vi "BuildRelease_FixAF2014.vi"(8 "error in (no error)":errorcluster, 11 "Array in":refnum<vi>[](array[refnum])) -> (0 "error out":errorcluster, 3 "Array out":refnum<vi>[](array[refnum]))   [LabVIEW 2020]
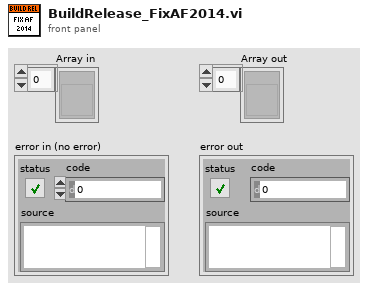
[diagram p1: front panel]
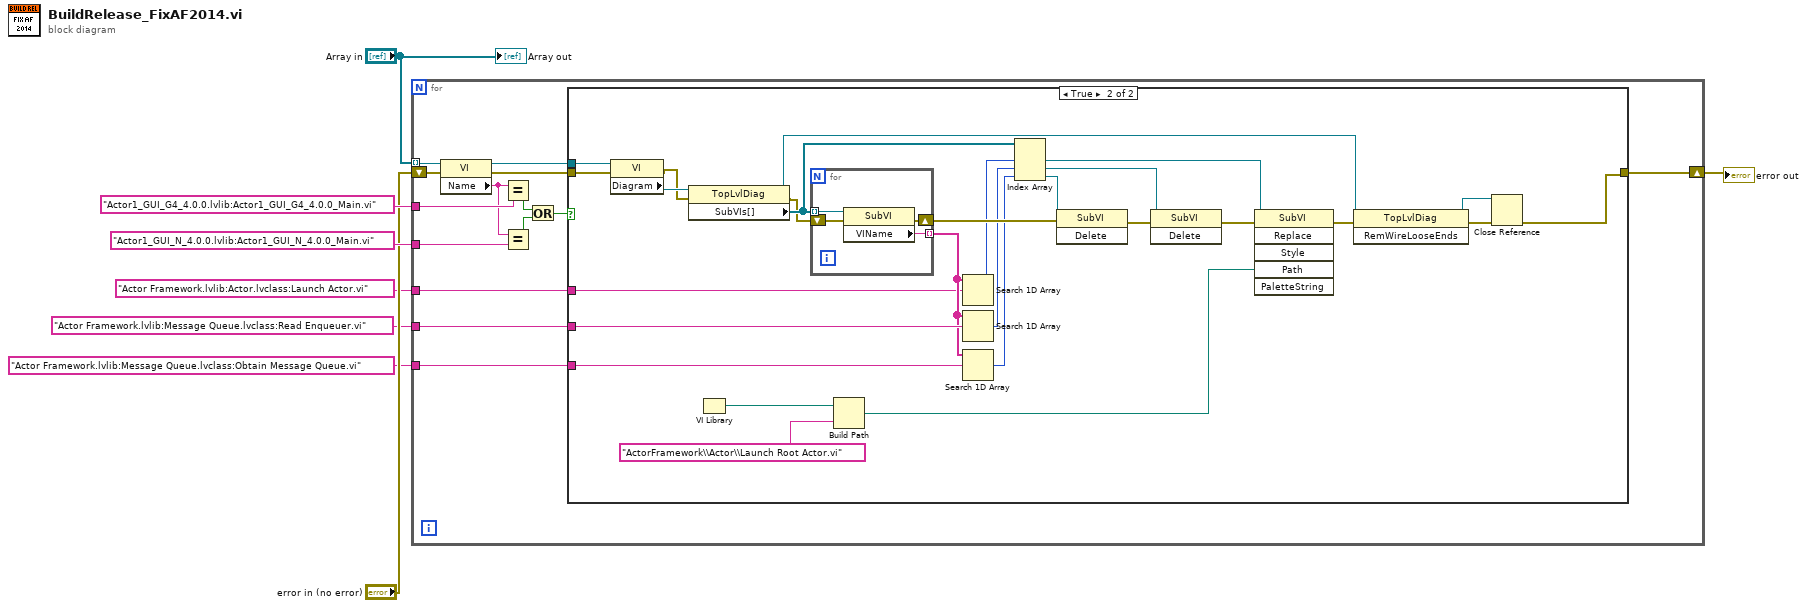
[diagram p0: block diagram]
diagram:
  n1 = for {
    tunnel: "Array in" -> [w22] mode=indexing
    tunnel: "Actor1_GUI_G4_4.0.0.lvlib:Actor1_GUI_G4_4.0.0_Main.vi" ("y") -> [w21]
    tunnel: "Actor1_GUI_N_4.0.0.lvlib:Actor1_GUI_N_4.0.0_Main.vi" ("y") -> [w19]
    shift-right: [w12] -> w4
    shift-left: "error in (no error)" -> [w13]
    tunnel: "Actor Framework.lvlib:Message Queue.lvclass:Obtain Message Queue.vi" ("y") -> [w11]
    tunnel: "Actor Framework.lvlib:Message Queue.lvclass:Read Enqueuer.vi" ("y") -> [w10]
    tunnel: "Actor Framework.lvlib:Actor.lvclass:Launch Actor.vi" ("y") -> [w9]
    n2 = property class="VI"(reference=w22, error in=w13) -> (reference out=w15:refnum<vi>, error out=w14:errorcluster, "Name"=w20:string)
    n3 = Equal?(x=w20, y=w21) -> (x = y?=w18:bool)
    n4 = Equal?(x=w20, y=w19) -> (x = y?=w17:bool)
    n5 = Or(x=w18, y=w17) -> (x .or. y?=w16:bool)
    n6 = case shown="True" w16 {
      tunnel: w15 -> [_ w50]
      tunnel: w14 -> [w23 w48]
      tunnel: [w23 w24] -> w12
      tunnel: w11 -> [_ w46]
      tunnel: w10 -> [_ w40]
      tunnel: w9 -> [_ w38]
      frame False {
      }
      frame True {
        n7 = property class="VI"(reference=w50, error in=w48) -> (error out=w47:errorcluster, "Diagram"=w49:refnum<vi>)  [unwired: 1 out]
        n8 = property class="TopLvlDiag"(reference=w49, error in=w47) -> (reference out=w27:refnum<vi>, error out=w44:errorcluster, "SubVIs[]"=w45:refnum<vi>[])
        n9 = VI Library() -> (path=w31:path)
        n10 = for {
          tunnel: w45 -> [w54] mode=indexing
          tunnel: [w53] -> w39 mode=indexing
          shift-right: [w51] -> w43
          shift-left: w44 -> [w52]
          n11 = property class="SubVI"(reference=w54, error in=w52) -> (error out=w51:errorcluster, "VIName"=w53:string)  [unwired: 1 out]
        }
        n12 = Build Path(base path=w31, name or relative path="ActorFramework\\Actor\\Launch Root Actor.vi") -> (appended path=w29:path)
        n13 = Search 1D Array(1D array=w39, element=w38) -> (index of element=w34:i32)  [unwired: 1 in]
        n14 = Search 1D Array(1D array=w39, element=w40) -> (index of element=w33:i32)  [unwired: 1 in]
        n15 = Search 1D Array(1D array=w39, element=w46) -> (index of element=w32:i32)  [unwired: 1 in]
        n16 = Index Array(array=w45, index #1=w34, index #2=w33, index #3=w32) -> (element #1=w35:refnum<vi>, element #2=w36:refnum<vi>, element #3=w42:refnum<vi>)
        n17 = invoke class="SubVI" method="Delete"(reference=w42, error in=w43) -> (error out=w41:errorcluster)  [unwired: 1 in, 2 out]
        n18 = invoke class="SubVI" method="Delete"(reference=w36, error in=w41) -> (error out=w37:errorcluster)  [unwired: 1 in, 2 out]
        n19 = invoke class="SubVI" method="Replace"(reference=w35, error in=w37, "Path"=w29) -> (error out=w28:errorcluster)  [unwired: 3 in, 5 out]
        n20 = invoke class="TopLvlDiag" method="RemWireLooseEnds"(reference=w27, error in=w28) -> (reference out=w25:refnum<vi>, error out=w26:errorcluster)  [unwired: 1 in, 1 out]
        n21 = Close Reference(reference=w25, error in (no error)=w26) -> (error out=w24:errorcluster)
      }
    }
  }
  "error out" <- w4
  "Array out" <- "Array in"
